vi "KepcoDCPwr Configure Voltage Mode.vi"(0 "VISA Session":refnum<visa-resource-name>, 1 "Transient Time (0.0005 seconds)":dbl=0.0005 format="%^.2e", 5 "Model In":string, 7 "Channel Name (\"\")":string, 9 "Mode (Fixed)":T1(ring), 11 "error in (no error)":errorcluster {"code" format="%.0x"}) -> (4 "VISA Session Out":refnum<visa-resource-name>, 6 "Model Out":string, 8 "channel name out (\"\")":string="\"\"" caption="channel name Out (\"\")", 15 "error out":errorcluster {"code" format="%.0x"})   [LabVIEW 2020]
doc: "This VI configures the Power supply operating mode.\n\nFixed - unit is outputing a single voltage and current setting\nTRAN - Transint operation, next setpoint will be applied for a period of time defined by the transient time setting.\nLIST - A list of some number of points will be executed.\n\nEXT - BOP and BIT devices only - enable external mode\nGAIN - BOP only - Enables Gain mode allowing external reference to be proportionally applied to ouput.\nPROT - BOP only- allows access the ot protecting settpoint valuse. \n Example CURR 10.1 is allowed and sets current setpoint to 10 but current protect to 10.1"
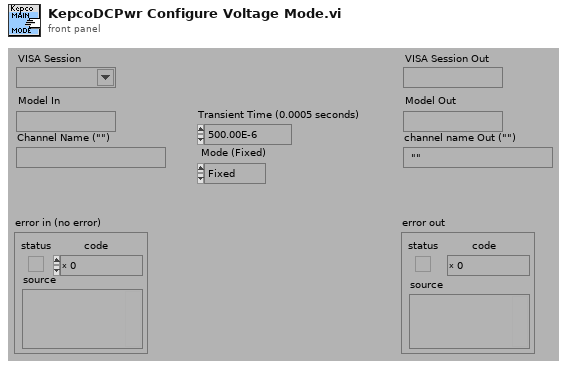
[diagram p1: front panel]
types:
  T1 = enum16{"Fixed", "List", "Transient", "External", "Gain", "Protect"}
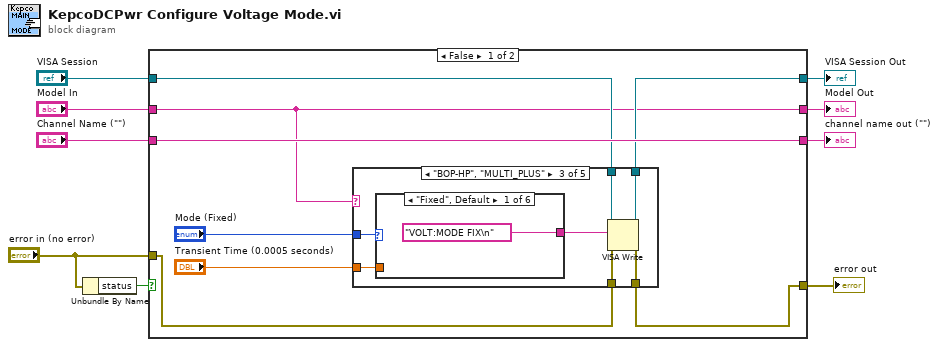
[diagram p0: block diagram]
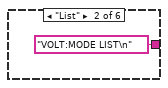
[diagram p4: hidden frame]
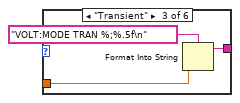
[diagram p5: hidden frame]
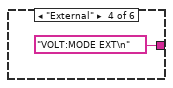
[diagram p6: hidden frame]
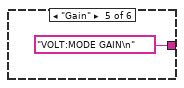
[diagram p7: hidden frame]
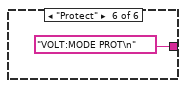
[diagram p8: hidden frame]
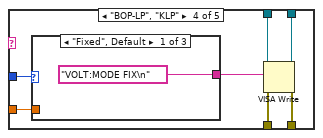
[diagram p9: hidden frame]
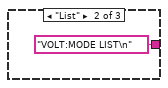
[diagram p10: hidden frame]
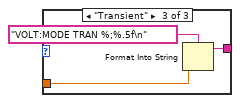
[diagram p11: hidden frame]
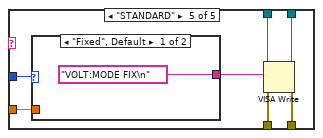
[diagram p12: hidden frame]
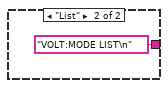
[diagram p13: hidden frame]
diagram:
  n1 = Unbundle By Name("error in (no error)") -> ("status"=w8:bool)
  n2 = case shown="False" w8 {
    tunnel: [w14 w61] -> w9
    tunnel: "error in (no error)" -> [w13 w61]
    tunnel: [w15 w60] -> w6
    tunnel: "VISA Session" -> [w16 w60]
    tunnel: "Model In" -> [w12 w59]
    tunnel: "Channel Name (\"\")" -> [w17 w58]
    tunnel: [w12 w59] -> w2
    tunnel: [w17 w58] -> w1
    frame False {
      n3 = case shown="\"BOP-HP\", \"MULTI_PLUS\"" w12 {
        tunnel: w13 -> [w19 w21 w28 w43 w55]
        tunnel: [w19 w21 w27 w42 w54] -> w14
        tunnel: w16 -> [w18 w20 w26 w41 w53]
        tunnel: [w18 w20 w25 w40 w52] -> w15
        tunnel: "Transient Time (0.0005 seconds)" -> [_ _ w24 w39 w51]
        tunnel: "Mode (Fixed)" -> [_ _ w22 w37 w49]
        frame "", Default {
        }
        frame "MULTI" {
        }
        frame "BOP-HP", "MULTI_PLUS" {
          n4 = case shown="\"Fixed\", Default" w22 {
            tunnel: w24 -> [_ _ w32 _ _ _]
            tunnel: ["VOLT:MODE FIX\n" "VOLT:MODE LIST\n" w31 "VOLT:MODE EXT\n" "VOLT:MODE GAIN\n" "VOLT:MODE PROT\n"] -> w23
            frame "Fixed", Default {
            }
            frame "List" {
            }
            frame "Transient" {
              n5 = Format Into String(format string="VOLT:MODE TRAN %;%.5f\n", w32) -> (resulting string=w31:string)  [unwired: 2 in, 1 out]
            }
            frame "External" {
            }
            frame "Gain" {
            }
            frame "Protect" {
            }
          }
          n6 = VISA Write(VISA resource name=w26, write buffer=w23, error in (no error)=w28) -> (VISA resource name out=w25:refnum<visa-resource-name>, error out=w27:errorcluster)  [unwired: 1 out]
        }
        frame "BOP-LP", "KLP" {
          n7 = case shown="\"Fixed\", Default" w37 {
            tunnel: w39 -> [_ _ w47]
            tunnel: ["VOLT:MODE FIX\n" "VOLT:MODE LIST\n" w46] -> w38
            frame "Fixed", Default {
            }
            frame "List" {
            }
            frame "Transient" {
              n8 = Format Into String(format string="VOLT:MODE TRAN %;%.5f\n", w47) -> (resulting string=w46:string)  [unwired: 2 in, 1 out]
            }
          }
          n9 = VISA Write(VISA resource name=w41, write buffer=w38, error in (no error)=w43) -> (VISA resource name out=w40:refnum<visa-resource-name>, error out=w42:errorcluster)  [unwired: 1 out]
        }
        frame "STANDARD" {
          n10 = case shown="\"Fixed\", Default" w49 {
            tunnel: w51 -> [_ _]
            tunnel: ["VOLT:MODE FIX\n" "VOLT:MODE LIST\n"] -> w50
            frame "Fixed", Default {
            }
            frame "List" {
            }
          }
          n11 = VISA Write(VISA resource name=w53, write buffer=w50, error in (no error)=w55) -> (VISA resource name out=w52:refnum<visa-resource-name>, error out=w54:errorcluster)  [unwired: 1 out]
        }
      }
    }
    frame True {
    }
  }
  "error out" <- w9
  "VISA Session Out" <- w6
  "channel name out (\"\")" <- w1
  "Model Out" <- w2
